vi "Write Text.vi"(8 "error in (no error)":errorcluster, 10 "Text":string, 11 "Text in":refnum<class "Text.lvclass">) -> (0 "error out":errorcluster, 3 "Text out":refnum<class "Text.lvclass">)   [LabVIEW 2015, in "LV Image Editor Framework.lvlib" / "Text.lvclass"]
uses:
  Text.lvclass
  Text.lvclass/Text.ctl
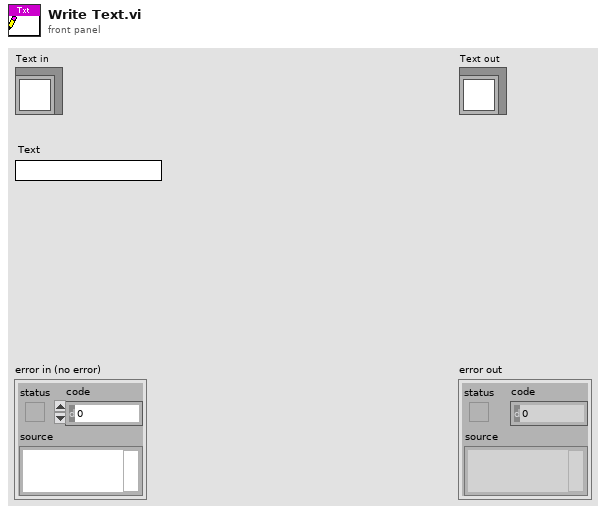
[diagram p1: front panel]
types:
  T1 = enum16{"User-specified Font", "Application Font", "System Font", "Dialog Font"}
  T2 = cluster{"Font Name:":string, "Size":i16, "Strikeout?":bool, "Italic?":bool, "Underline?":bool, "Outline?":bool, "Shadow?":bool, "Bold?":bool}
  T3 = cluster{"left":i16, "top":i16, "right":i16, "bottom":i16}
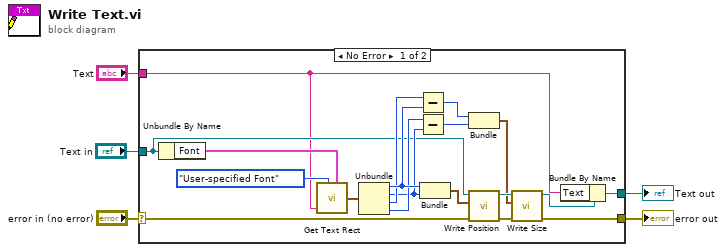
[diagram p0: block diagram]
diagram:
  n1 = case shown="No Error" "error in (no error)" {
    selector: "error in (no error)" -> [w9 w25]
    tunnel: [w7 w25] -> w4
    tunnel: [w24 w26] -> w2
    tunnel: "Text in" -> [w14 w26]
    tunnel: "Text" -> [w6 _]
    frame No Error {
      n2 = Unbundle By Name(w14) -> ("Font"=w20:T2)
      n3 = call <vilib>:"Get Text Rect.vi"("desired font(Application)"=T1."User-specified Font", "text"=w6, "[user-specified font]"=w20) -> ("rect"=w19:T3)  [unwired: 6 in]
      n4 = Unbundle(w19) -> ("left"=w23:i16, "top"=w16:i16, "right"=w18:i16, "bottom"=w17:i16)
      n5 = Subtract(x=w18, y=w23) -> (x-y=w22:i16)
      n6 = Subtract(x=w17, y=w16) -> (x-y=w15:i16)
      n7 = Bundle("left"=w23, "top"=w16) -> (w11:cluster{"left":i16, "top":i16})  [unwired: 1 in]
      n8 = Bundle(w22, w15) -> (w10:cluster{i16, i16})  [unwired: 1 in]
      n9 = call-dynamic "Write Position.vi"("error in (no error)"=w9, "Position"=w11, "Shape in"=w14) -> ("error out"=w8:errorcluster, "Shape out"=w13:refnum<class "Text.lvclass">)  [unwired: 7 in]
      n10 = call-dynamic "Write Size.vi"("error in (no error)"=w8, "Size"=w10, "Shape in"=w13) -> ("error out"=w7:errorcluster, "Shape out"=w12:refnum<class "Text.lvclass">)  [unwired: 7 in]
      n11 = Bundle By Name(cluster=w12, "Text"=w6) -> (w24:refnum<class "Text.lvclass">)
    }
    frame Error {
    }
  }
  "error out" <- w4
  "Text out" <- w2
